vi "数据摘要提取.vi"(9 "数据索引":i32[](array[numeric]), 11 "数组输入":T1[](array[typedef])) -> (0 "删除？":bool[](array[boolean]), 1 "数据摘要":string[][](array[string]), 3 "数组输出":T1[](array[typedef]))   [LabVIEW 2020]
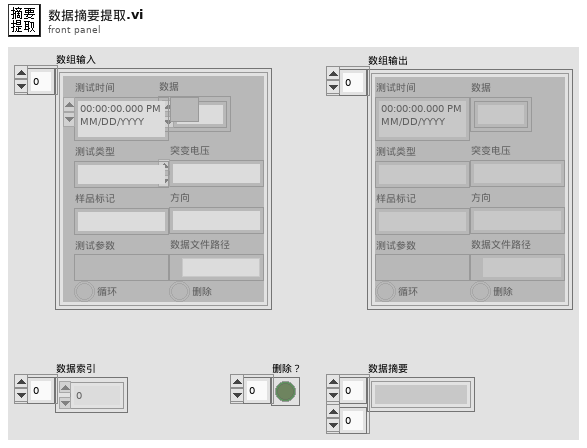
[diagram p1: front panel]
types:
  T1 = typedef "测试数据类型.ctl" = cluster{"测试时间":timestamp, "测试类型":string, "样品标记":string, "测试参数":variant, "循环":bool, "数据":dbl[][], "删除":bool, "突变电压":i32, "方向":string, "数据文件路径":path}
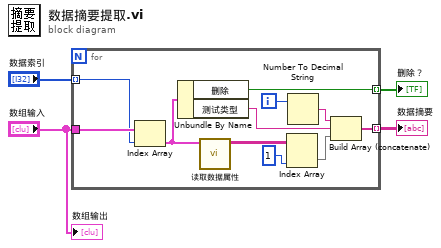
[diagram p0: block diagram]
diagram:
  n1 = for {
    tunnel: "数组输入" -> [w15]
    tunnel: "数据索引" -> [w14] mode=indexing
    tunnel: [w5] -> w2 mode=indexing
    tunnel: [w7] -> w1 mode=indexing
    i -> [w6]
    n2 = Index Array(array=w15, index=w14) -> (element=w11:T1)
    n3 = Unbundle By Name(w11) -> ("删除"=w5:bool, "测试类型"=w9:string)
    n4 = call "读取数据属性.vi"("测试数据"=w11) -> ("数据属性"=w13:string[][])  [unwired: 10 in]
    n5 = Index Array(array=w13, index (col)=1 ("禁用的索引 (列)")) -> (element=w8:string[])  [unwired: 1 in]
    n6 = Number To Decimal String(number=w6) -> (decimal integer string=w10:string)  [unwired: 1 in]
    n7 = Build Array (concatenate)(w10, w9, w8) -> (w7:string[])
  }
  "数据摘要" <- w1
  "删除？" <- w2
  "数组输出" <- "数组输入"
